vi "parseError.vi"(1 "Error In":errorcluster, 10 "ump dll return value (<0 is error)":i32) -> (16 "Sucessful lib call?":bool, 21 "Error Out":errorcluster)   [LabVIEW 2016, in "OSB_uMp_library.lvlib"]
doc: "Check return value of library call (dll call).\n\nCreates a LabVIEW error cluster if return value is error"
uses:
  OSB_uMp_library.lvlib
panel:
  # "By Stuart Box at OxSyBio Ltd, 2017\n\nThis software is provided WITHOUT ANY WARRANTY; without even the implied warranty of MERCHANTABILITY or FITNESS FOR A PARTICULAR PURPOSE.\n\ninfo@oxsybio.com\n\nOxSyBio Ltd, The Walbrook Building, 25 Walbrook, London, EC4N 8AF"
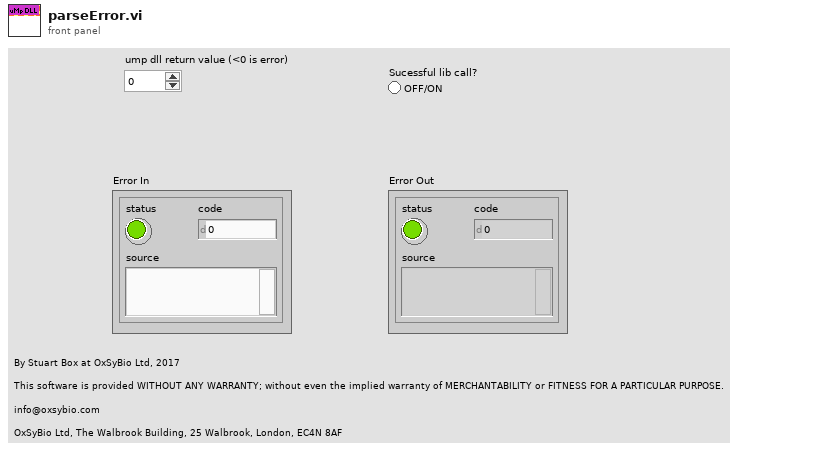
[diagram p1: front panel]
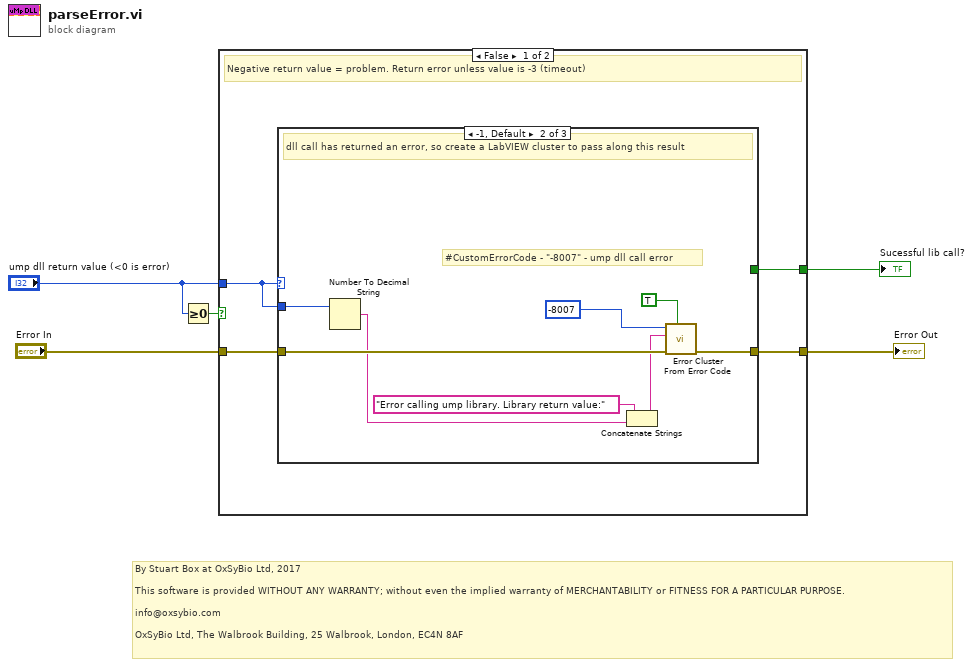
[diagram p0: block diagram]
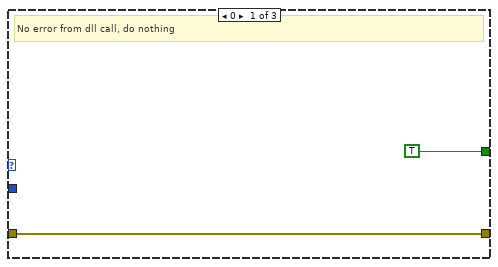
[diagram p2: hidden frame]
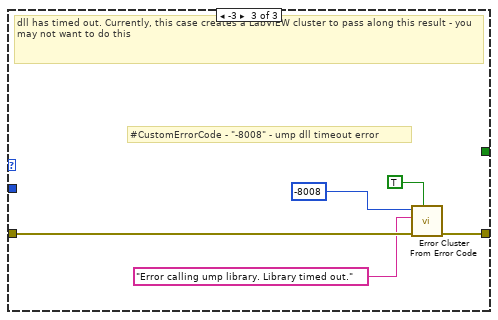
[diagram p3: hidden frame]
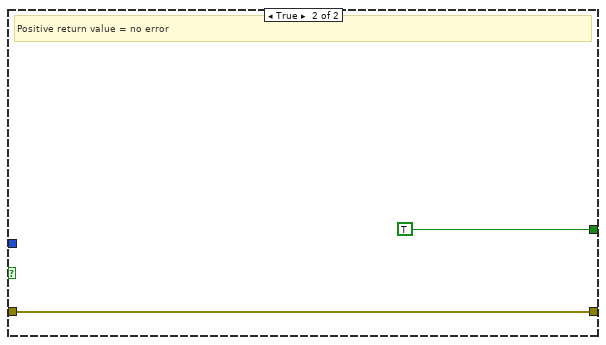
[diagram p4: hidden frame]
diagram:
  # "By Stuart Box at OxSyBio Ltd, 2017\n\nThis software is provided WITHOUT ANY WARRANTY; without even the implied warranty of MERCHANTABILITY or FITNESS FOR A PARTICULAR PURPOSE.\n\ninfo@oxsybio.com\n\nOxSyBio Ltd, The Walbrook Building, 25 Walbrook, London, EC4N 8AF"
  n1 = Greater Or Equal To 0?(x="ump dll return value (<0 is error)") -> (x >= 0?=w1:bool)
  n2 = case shown="False" w1 {
    tunnel: "Error In" -> [w9 w26]
    tunnel: [w8 w26] -> w4
    tunnel: "ump dll return value (<0 is error)" -> [w7 _]
    tunnel: [w6 TRUE] -> w3
    frame False {
      # "Negative return value = problem. Return error unless value is -3 (timeout)"
      n3 = case shown="-1, Default" w7 {
        tunnel: w9 -> [w11 w17 w22]
        tunnel: [w11 w16 w21] -> w8
        tunnel: w7 -> [_ w15 _]
        tunnel: [TRUE _ _] -> w6
        frame 0 {
          # "No error from dll call, do nothing"
        }
        frame -1, Default {
          # "#CustomErrorCode - \"-8007\" - ump dll call error"
          # "dll call has returned an error, so create a LabVIEW cluster to pass along this result"
          n4 = Number To Decimal String(number=w15) -> (decimal integer string=w12:string)  [unwired: 1 in]
          n5 = Concatenate Strings("Error calling ump library. Library return value:" ("error message (\"\")"), w12) -> (w13:string)
          n6 = call <vilib>:"Error Cluster From Error Code.vi"("show call chain? (False)"=TRUE, "error in (no error)"=w17, "error message (\"\")"=w13, "error code (0)"=-8007) -> ("error out"=w16:errorcluster)  [unwired: 5 in]
        }
        frame -3 {
          # "#CustomErrorCode - \"-8008\" - ump dll timeout error"
          # "dll has timed out. Currently, this case creates a LabVIEW cluster to pass along this result - you may not want to do this"
          n7 = call <vilib>:"Error Cluster From Error Code.vi"("show call chain? (False)"=TRUE, "error in (no error)"=w22, "error message (\"\")"="Error calling ump library. Library timed out." ("error message (\"\")"), "error code (0)"=-8008) -> ("error out"=w21:errorcluster)  [unwired: 5 in]
        }
      }
    }
    frame True {
      # "Positive return value = no error"
    }
  }
  "Error Out" <- w4
  "Sucessful lib call?" <- w3
